vi "graph 1.vi"() -> ()   [LabVIEW 2019]
panel:
  out "graph Y (deux courbes)\ncos et sin en fonction de l'indice":dbl[][](graph)
  out "Graph Y (une courbe)\ncos en fonction de l'indice":dbl[](graph)
  out "XY Graph\ncos(x) en fonction de x":cluster{dbl[], dbl[]}(graph)
  out "graph déroulant":dbl(graph)
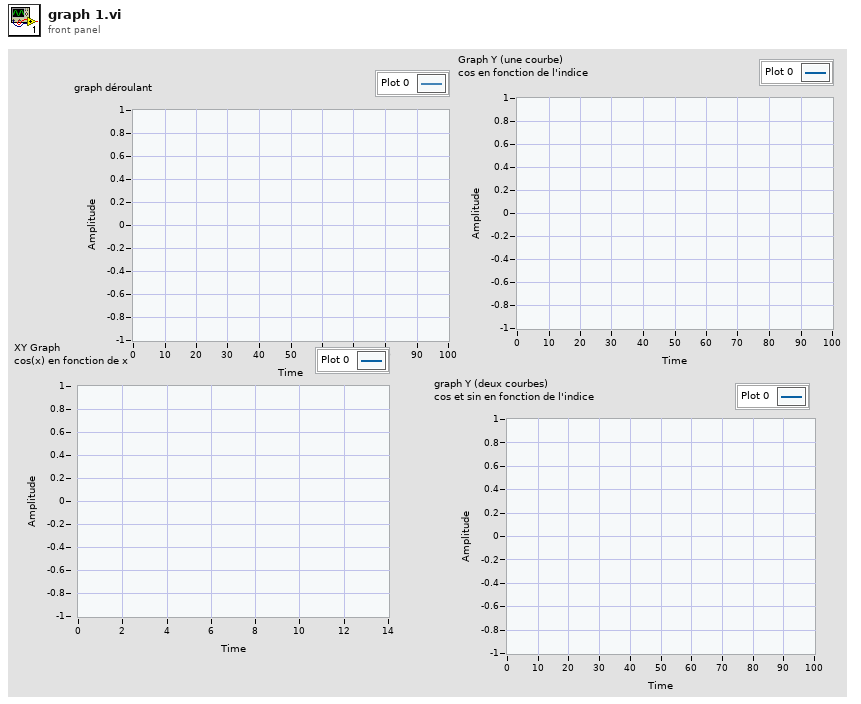
[diagram p1: front panel]
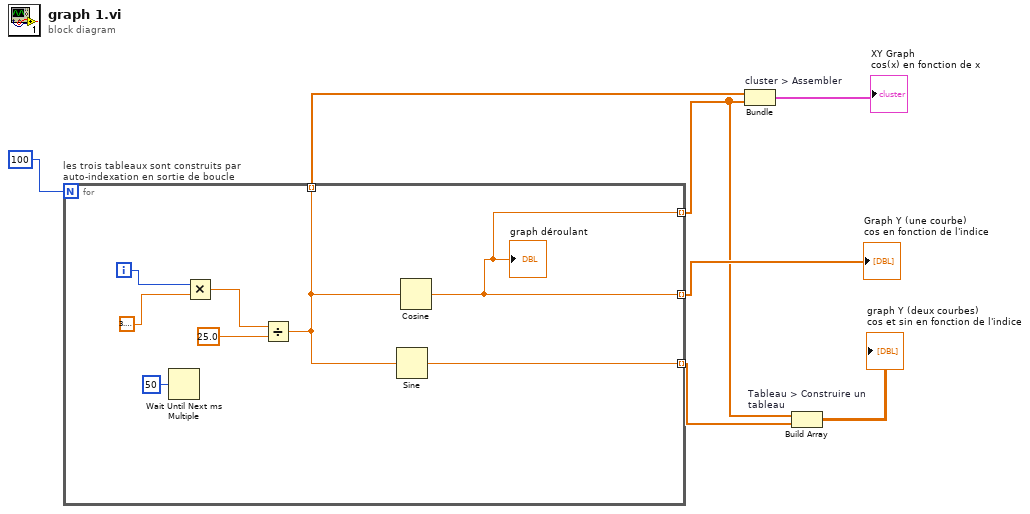
[diagram p0: block diagram]
diagram:
  n1 = for "les trois tableaux sont construits par auto-indexation en sortie de boucle" {
    N: 100 -> [_]
    tunnel: [w9] -> w4 mode=indexing
    tunnel: [w10] -> w2 mode=indexing
    tunnel: [w9] -> w3 mode=indexing
    tunnel: [w8] -> w6 mode=indexing
    i -> [w15]
    n2 = Wait Until Next ms Multiple(millisecond multiple=50) -> ()  [unwired: 1 out]
    n3 = Multiply(x=w15, y=3.141592653589793) -> (x*y=w13:dbl)
    n4 = Divide(x=w13, y=25.0) -> (x/y=w8:dbl)
    n5 = Sine(x=w8) -> (sin(x)=w10:dbl)
    n6 = Cosine(x=w8) -> (cos(x)=w9:dbl)
    "graph déroulant" <- w9
  }
  "Graph Y (une courbe)\ncos en fonction de l'indice" <- w4
  n7 = Bundle "cluster > Assembler"(w6, w3) -> (→"XY Graph\ncos(x) en fonction de x":cluster{dbl[], dbl[]})  [unwired: 1 in]
  n8 = Build Array "Tableau > Construire un tableau"(w3, w2) -> (→"graph Y (deux courbes)\ncos et sin en fonction de l'indice":dbl[][])
